vi "Main (RT).vi"() -> ()   [LabVIEW 2016]
uses:
  <vilib>/rvi/interface/nirviReadWriteControl/nirviReadWriteControl.xnode
  <vilib>/rvi/interface/nirviCloseFPGA/nirviCloseFPGA.xnode
  <vilib>/rvi/interface/nirviOpenFPGA/nirviOpenFPGA.xnode
  FPGA Bitfiles/DHT22Sensor_FPGATarget_Example-DHT22(FP_mGMjaUny0lU.lvbitx
  DHT22 Library/Example - DHT22 (FPGA).vi
  <vilib>/rvi/interface/Simulation/niFpgaSimulationCallBeginRW.vi
  <vilib>/rvi/errors/niLvFpgaAdjustHostInterfaceError.vi
  <vilib>/FPGAPlugInAG/Dynamic/niLvFpga_Close_Dynamic.vi
panel:
  out "DHT 22 - error out":errorcluster
  out "Temperature (°F)":dbl(slide) scale=0.0..100.0
  out "Humidity (%)":dbl(slide) scale=0.0..100.0
  out "Temperature (°C)":dbl(slide) scale=0.0..100.0
  out "error out":errorcluster
  in  "Stop Button":bool
  out "Chart":cluster{dbl, dbl}(graph)
  # "Error -8001: Checksum Error\nError- 8002: Timeout Error"
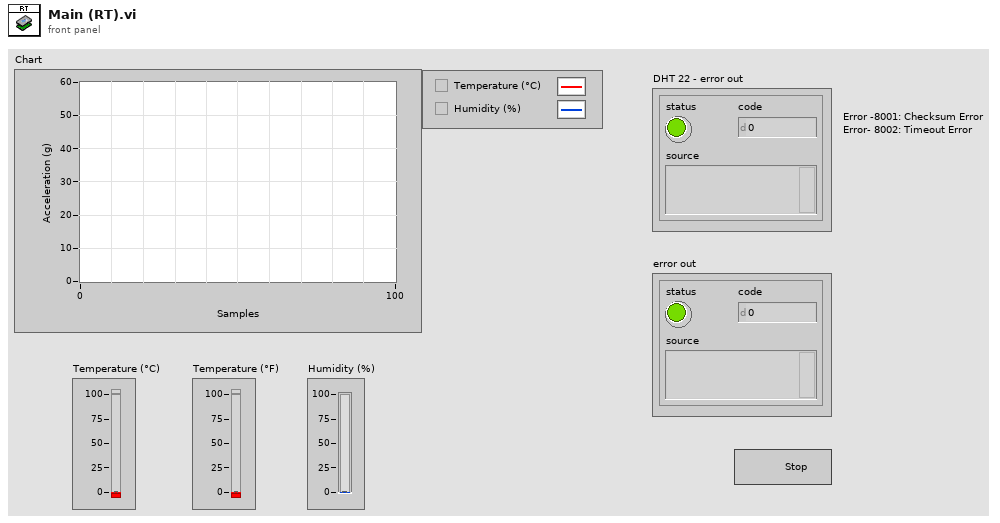
[diagram p1: front panel]
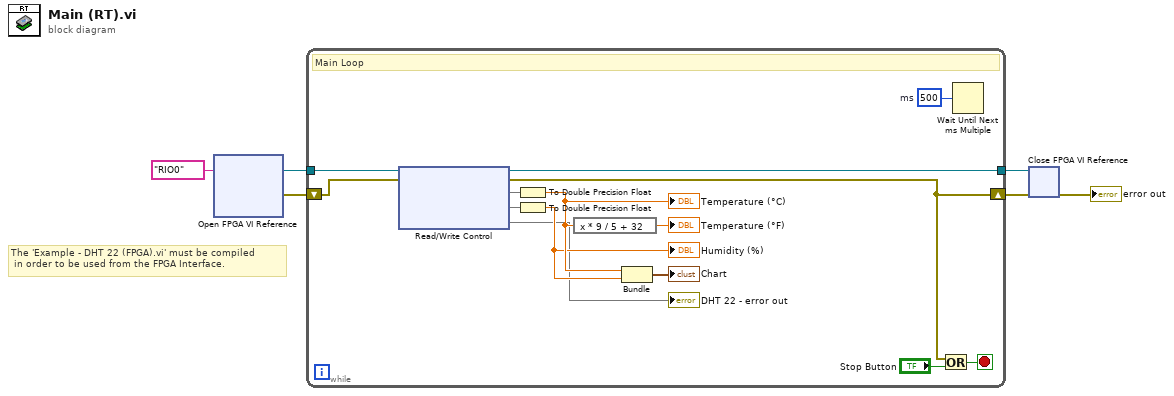
[diagram p0: block diagram]
diagram:
  # "The 'Example - DHT 22 (FPGA).vi' must be compiled\n in order to be used from the FPGA Interface."
  n1 = xnode "Open FPGA VI Reference"("resource name"=tag "RIO0") -> ("FPGA VI Reference Out"=w3:refnum<k20>, "error out"=w2:errorcluster)  [unwired: 1 in]
  n2 = while {
    tunnel: w3 -> [w18]
    tunnel: [w16] -> w6
    shift-right: [w14] -> w5
    shift-left: w2 -> [w10]
    stop <- w19 stop-if-true
    w17 = u32 500  # ms
    # "Main Loop"
    n3 = xnode "Read/Write Control"("FPGA VI Reference In"=w18, "error in"=w10) -> ("FPGA VI Reference Out"=w16:refnum<k20>, "error out"=w14:errorcluster, "Temperature (°C)"=w13, "Humidity (%)"=w11, "error out"=→"DHT 22 - error out")
    n4 = To Double Precision Float(number=w13) -> (double precision float=w9:dbl)
    "Temperature (°C)" <- w9
    n5 = To Double Precision Float(number=w11) -> (double precision float=w8:dbl)
    "Humidity (%)" <- w8
    n6 = expression code="x * 9 / 5 + 32"(w9) -> (→"Temperature (°F)":dbl)
    n7 = Bundle(w9, w8) -> (→"Chart":cluster{dbl, dbl})  [unwired: 1 in]
    n8 = Or(x=w14, y="Stop Button") -> (x .or. y?=w19:bool)
    n9 = Wait Until Next ms Multiple(millisecond multiple=w17) -> ()  [unwired: 1 out]
  }
  n10 = xnode "Close FPGA VI Reference"("FPGA VI Reference In"=w6, "error in"=w5) -> ("error out"=→"error out":errorcluster)
